vi "GEvt-Generate Module Destroyed Log.vi"(0 "CSM Global Log Event":refnum<user-event>, 6 "Name(\"\" to use uuid)":string, 7 "Enable?":bool, 10 "CSM:LogFilter.lvclass":refnum<class "LogFilter.lvclass">) -> (14 "CSM Global Log Event out":refnum<user-event>, 16 "event data":T1={"Name(\"\" to use uuid)"="", "Current State"="", "Arguments"="", "Source Message"={"‘State"="", "’Arguments"="", "’Error"={"status"=FALSE, "code"=0, "source"=""}}, "Source Module"="", "Complete(T)/Start(F)"=FALSE, "LogType"=enum."State Change"})   [LabVIEW 2020, in "Communicable State Machine.lvlib"]
uses:
  Communicable State Machine.lvlib
  _CSM_GlobalLog_MSG.ctl
  _CSM_Response Source Message.ctl
  _CSM_GlobalLog_MSG_TYPE.ctl
  LogFilter.lvclass
  Filter Check.vi
  Group Check - CSM.vi
  Group Check - LogType.vi
  Group Check - State.vi
  CSM Check - LogType.vi
  CSM Check - State.vi
  CSM Check - StateType.vi
  Group Check - StateType.vi
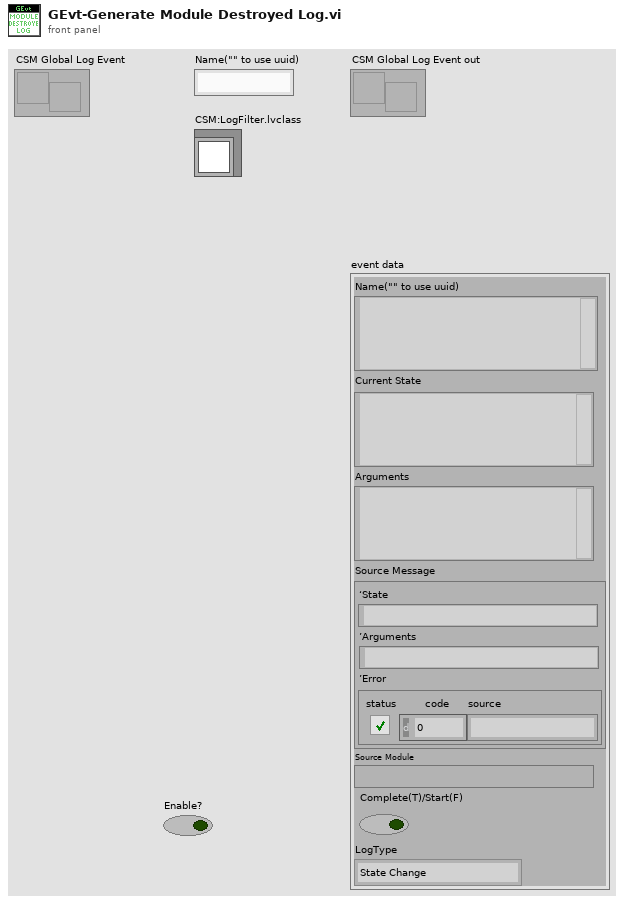
[diagram p1: front panel]
types:
  T1 = typedef "Communicable State Machine.lvlib/_CSM_GlobalLog_MSG.ctl" = cluster{"Name(\"\" to use uuid)":string, "Current State":string, "Arguments":string, "Source Message":T2, "Source Module":string, "Complete(T)/Start(F)":bool, "LogType":T3}
  T2 = typedef "Communicable State Machine.lvlib/_CSM_Response Source Message.ctl" = cluster{"‘State":string, "’Arguments":string, "’Error":errorcluster}
  T3 = typedef "Communicable State Machine.lvlib/_CSM_GlobalLog_MSG_TYPE.ctl" = enum16{"User Log", "State Change", "Status", "Interrupt", "Register", "Unregister", "Error Log", "Module Created", "Module Destroyed"}
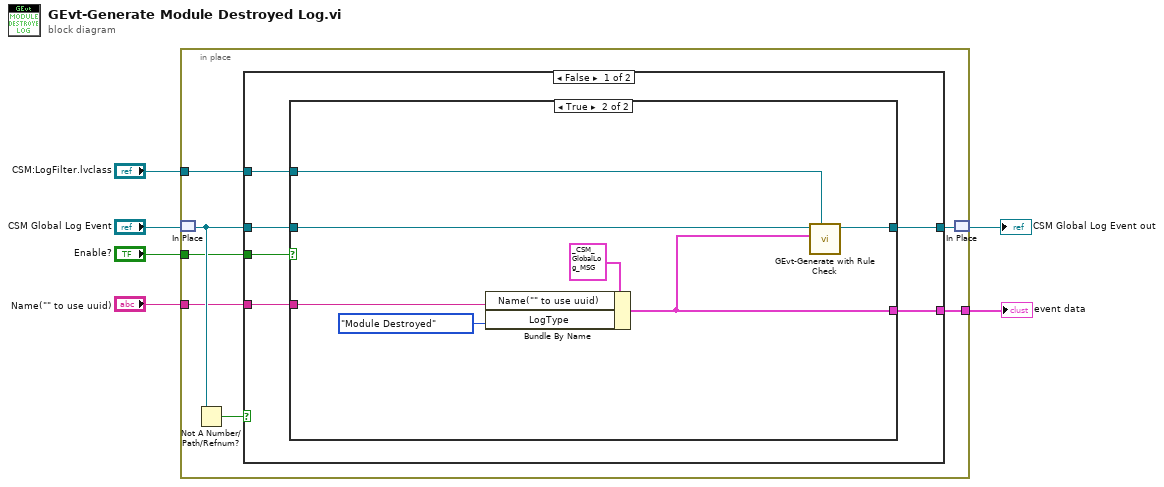
[diagram p0: block diagram]
diagram:
  n1 = in-place {
    in-place-border: [w10] -> w4
    in-place-border: "Enable?" -> [w9]
    in-place-border: "Name(\"\" to use uuid)" -> [w8]
    in-place-border: "CSM:LogFilter.lvclass" -> [w7]
    n2 = in-place-match #1("CSM Global Log Event") -> (w12:refnum<user-event>)
    n3 = Not A Number/Path/Refnum?(number/path/refnum=w12) -> (NaN/Path/Refnum?=w13:bool)
    n4 = case shown="False" w13 {
      tunnel: w12 -> [w19 w28]
      tunnel: [w18 w28] -> w11
      tunnel: [w17 _] -> w10
      tunnel: w9 -> [w16 _]
      tunnel: w8 -> [w15 _]
      tunnel: w7 -> [w14 _]
      frame False {
        n5 = case shown="True" w16 {
          tunnel: w19 -> [w20 w27]
          tunnel: [w20 w26] -> w18
          tunnel: [_ w22] -> w17
          tunnel: w15 -> [_ w23]
          tunnel: w14 -> [_ w21]
          frame False {
          }
          frame True {
            n6 = Bundle By Name(cluster=T1 {"Name(\"\" to use uuid)"="", "Current State"="", "Arguments"="", "Source Message"={"‘State"="", "’Arguments"="", "’Error"={"status"=FALSE, "code"=0, "source"=""}}, "Source Module"="", "Complete(T)/Start(F)"=FALSE, "LogType"=enum."State Change"} ("event data"), "Name(\"\" to use uuid)"=w23, "LogType"=_CSM_GlobalLog_MSG_TYPE."Module Destroyed" ("Type")) -> (w22:T1)
            n7 = call "GEvt-Generate with Rule Check.vi"("LogFilter in"=w21, "event data"=w22, "CSM Global Log Event in"=w27) -> ("CSM Global Log Event out"=w26:refnum<user-event>)  [unwired: 8 in]
          }
        }
      }
      frame True {
      }
    }
    n8 = in-place-match #1(w11) -> (→"CSM Global Log Event out":refnum<user-event>)
  }
  "event data" <- w4
